vi "dither18bitTo16bit.vi"(11 "input":fxp<+/-,18,16>) -> (3 "output":cluster{i16, i16})   [LabVIEW 2016]
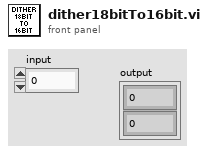
[diagram p1: front panel]
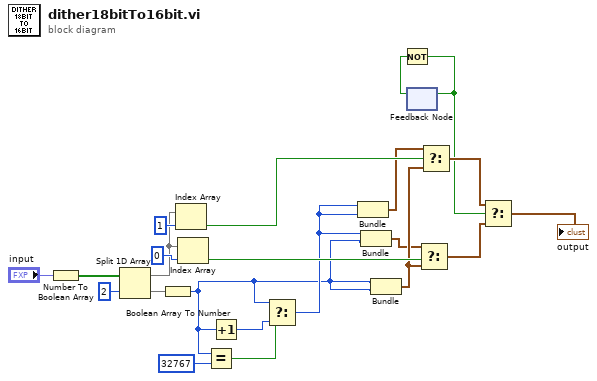
[diagram p0: block diagram]
diagram:
  n1 = Number To Boolean Array(number="input") -> (Boolean array=w4:bool[])
  n2 = Split 1D Array(array=w4, index=2) -> (first subarray=w16:bool[], second subarray=w7:bool[])
  n3 = Boolean Array To Number(Boolean array=w7) -> (number=w2:i16)
  n4 = Index Array(array=w16, index=1) -> (element=w18:bool)
  n5 = Index Array(array=w16, index=0) -> (element=w17:bool)
  n6 = Equal?(x=w2, y=i16 32767) -> (x = y?=w3:bool)
  n7 = Increment(x=w2) -> (x+1=w6:i16)
  n8 = Select(t=w2, s=w3, f=w6) -> (s? t:f=w5:i16)
  n9 = Bundle(w5, w5) -> (w9:cluster{i16, i16})  [unwired: 1 in]
  n10 = Bundle(w5, w2) -> (w10:cluster{i16, i16})  [unwired: 1 in]
  n11 = Bundle(w2, w2) -> (w11:cluster{i16, i16})  [unwired: 1 in]
  n12 = feedback #1() -> (w13:bool)  [unwired: 1 in]
  n13 = Not(x=w13) -> (.not. x?=w12:bool)
  n14 = feedback-in #1(w12) -> ()
  n15 = Select(t=w10, s=w17, f=w11) -> (s? t:f=w15:cluster{i16, i16})
  n16 = Select(t=w9, s=w18, f=w11) -> (s? t:f=w14:cluster{i16, i16})
  n17 = Select(t=w14, s=w12, f=w15) -> (s? t:f=→"output":cluster{i16, i16})
